vi "ObstacleBallRadius.vi"(9 "Goal":dbl[](array[numeric]), 10 "Initial State":dbl[](array[numeric]), 11 "ball":dbl[](array[numeric])) -> (2 "obstacle enemy radius":dbl)   [LabVIEW 2020]
uses:
  <vilib>/Analysis/_algsub.llb/Real Vector Norm.vi
  <vilib>/Analysis/NI_AALPro.lvlib
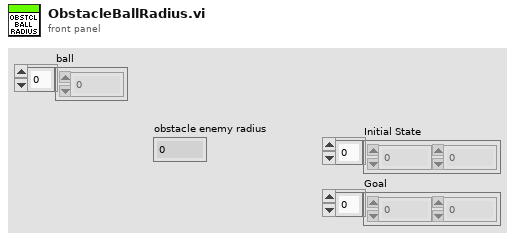
[diagram p1: front panel]
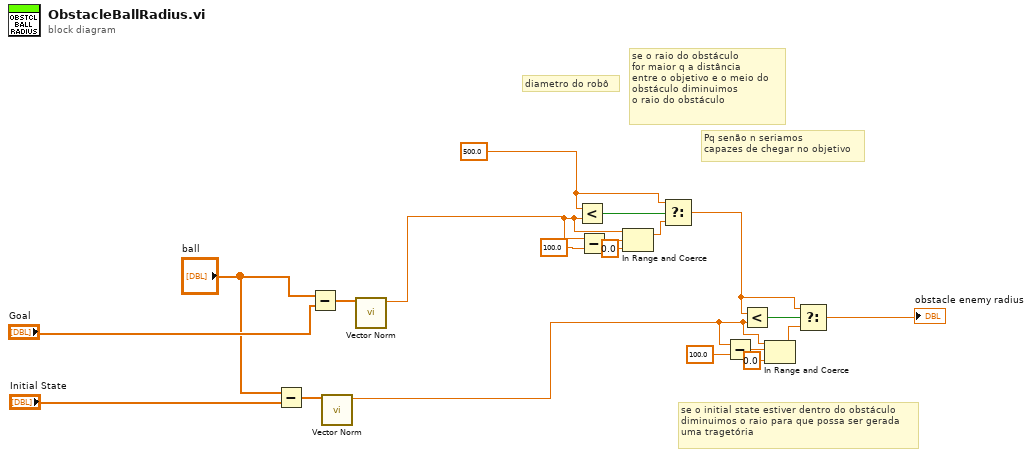
[diagram p0: block diagram]
diagram:
  w10 = 500.0 ("x")
  # "se o initial state estiver dentro do obstáculo\ndiminuimos o raio para que possa ser gerada\numa tragetória"
  # "diametro do robô"
  # "Pq senão n seriamos\ncapazes de chegar no objetivo"
  # "se o raio do obstáculo\nfor maior q a distância \nentre o objetivo e o meio do \nobstáculo diminuimos \no raio do obstáculo"
  n1 = Subtract(x="ball", y="Initial State") -> (x-y=w17:dbl[])
  n2 = Subtract(x="ball", y="Goal") -> (x-y=w20:dbl[])
  n3 = call-poly <vilib>:"Vector Norm.vi"("Input Vector"=w17) -> ("norm"=w3:dbl)  [unwired: 9 in, 1 out]
  n4 = call-poly <vilib>:"Vector Norm.vi"("Input Vector"=w20) -> ("norm"=w8:dbl)  [unwired: 9 in, 1 out]
  n5 = Less?(x=w10, y=w8) -> (x < y?=w19:bool)
  n6 = Subtract(x=w8, y=100.0) -> (x-y=w9:dbl)
  n7 = In Range and Coerce(upper limit=w8, x=w9, lower limit=0.0) -> (coerced(x)=w6:dbl)  [unwired: 1 out]
  n8 = Select(t=w10, s=w19, f=w6) -> (s? t:f=w13:dbl)
  n9 = Subtract(x=w3, y=100.0) -> (x-y=w4:dbl)
  n10 = Less?(x=w13, y=w3) -> (x < y?=w15:bool)
  n11 = In Range and Coerce(upper limit=w3, x=w4, lower limit=0.0) -> (coerced(x)=w2:dbl)  [unwired: 1 out]
  n12 = Select(t=w13, s=w15, f=w2) -> (s? t:f=→"obstacle enemy radius":dbl)
